vi "sub_Ready.vi"(8 "error in":errorcluster caption="에러 입력", 11 "Wash Options":refnum<vi>) -> (0 "error out":errorcluster caption="에러 출력")   [LabVIEW 2017]
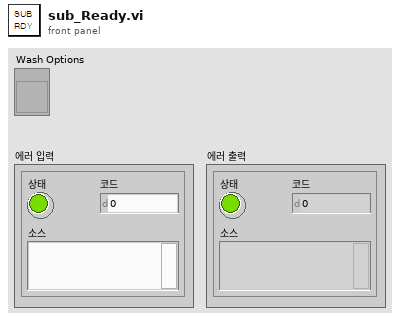
[diagram p1: front panel]
types:
  T1 = enum8{"Enabled", "Disabled", "Disabled and Grayed Out"}
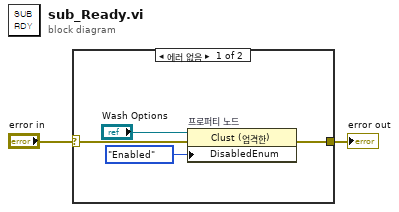
[diagram p0: block diagram]
diagram:
  n1 = case shown="에러 없음" "error in" {
    selector: "error in" -> [w5 w7]
    tunnel: [w6 w7] -> w1
    frame No Error {
      n2 = property on="프로퍼티 노드" class="Clust (엄격한)"(reference="Wash Options", error in=w5, "DisabledEnum"=T1."Enabled" ("비활성화")) -> (error out=w6:errorcluster)  [unwired: 1 out]
    }
    frame Error {
    }
  }
  "error out" <- w1
